vi "UI Events On.vi"(8 "error in (no error)":errorcluster, 10 "UI Events":T1, 11 "I_UI_Events in":refnum<class "I_UI_Events.lvclass">) -> (0 "error out":errorcluster, 3 "I_UI_Events out":refnum<class "I_UI_Events.lvclass">)   [LabVIEW 2020, in "Actor_UI_Template.lvlib" / "I_UI_Events.lvclass"]
uses:
  I_UI_Events.lvclass
  UI Event Enum.ctl
  Actor_UI_Template.lvlib
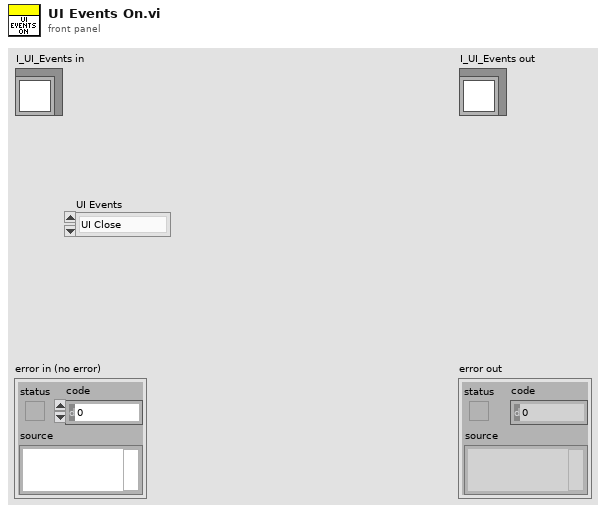
[diagram p1: front panel]
types:
  T1 = typedef "Actor_UI_Template.lvlib/UI Event Enum.ctl" = enum16{"UI Close"}
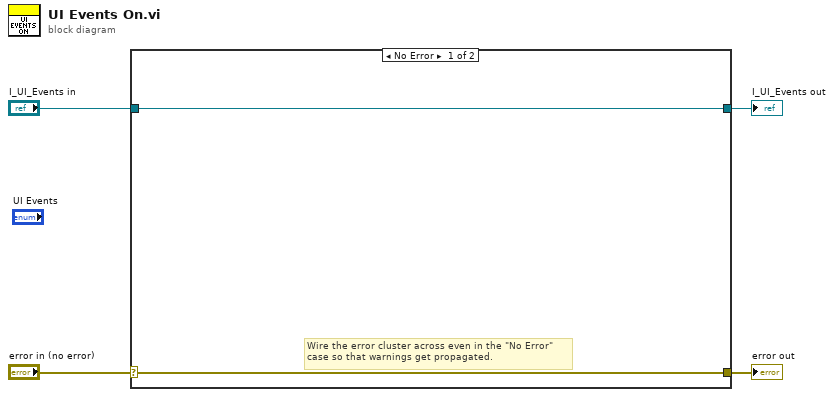
[diagram p0: block diagram]
diagram:
  n1 = case shown="No Error" "error in (no error)" {
    selector: "error in (no error)" -> [w5 w8]
    tunnel: [w5 w8] -> w3
    tunnel: [w6 w7] -> w1
    tunnel: "I_UI_Events in" -> [w6 w7]
    frame No Error {
      # "Wire the error cluster across even in the \"No Error\"\ncase so that warnings get propagated."
    }
    frame Error {
    }
  }
  "error out" <- w3
  "I_UI_Events out" <- w1
